vi "Frequency.vi"(8 "Samples per calculation":i32, 11 "Input waveform":waveform(dbl)) -> (3 "Frequency waveform":waveform(dbl))   [LabVIEW 2019]
uses:
  <vilib>/measure/mascope.llb/Pulse Measurements 1 chan.vi
  <vilib>/measure/NI_MAPro.lvlib
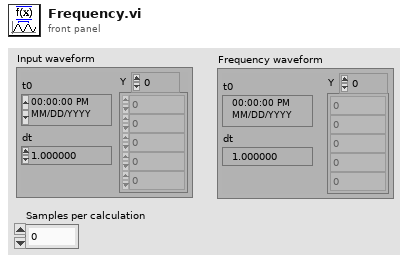
[diagram p1: front panel]
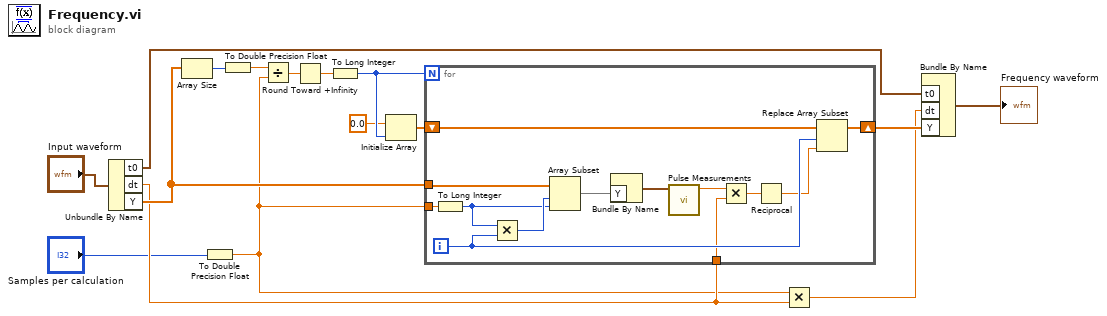
[diagram p0: block diagram]
diagram:
  n1 = Unbundle By Name("Input waveform") -> ("t0"=w5:timestamp, "dt"=w3:dbl, "Y"=w11:dbl[])
  n2 = Array Size(array=w11) -> (size(s)=w12:i32)
  n3 = To Double Precision Float(number="Samples per calculation") -> (double precision float=w1:dbl)
  n4 = To Double Precision Float(number=w12) -> (double precision float=w13:dbl)
  n5 = Divide(x=w13, y=w1) -> (x/y=w15:dbl)
  n6 = Round Toward +Infinity(x=w15) -> (ceil(x): smallest int >= x=w14:dbl)
  n7 = To Long Integer(number=w14) -> (32bit integer=w10:i32)
  n8 = Initialize Array(0.0 ("element"), w10) -> (w9:dbl[])
  n9 = for {
    N: w10 -> [_]
    tunnel: w11 -> [w28]
    tunnel: w1 -> [w26]
    shift-right: [w21] -> w6
    shift-left: w9 -> [w23]
    tunnel: w3 -> [w19]
    i -> [w22]
    n10 = To Long Integer(number=w26) -> (32bit integer=w24:i32)
    n11 = Multiply(x=w24, y=w22) -> (x*y=w25:i32)
    n12 = Array Subset(array=w28, index=w25, length=w24) -> (w27:dbl[])
    n13 = Bundle By Name("Y"=w27) -> (w29:waveform(dbl))  [unwired: 1 in]
    n14 = call-poly <vilib>:"Pulse Measurements.vi"("signal in"=w29) -> ("period"=w20:dbl)  [unwired: 6 in, 4 out]
    n15 = Multiply(x=w20, y=w19) -> (x*y=w18:dbl)
    n16 = Reciprocal(x=w18) -> (1/x=w17:dbl)
    n17 = Replace Array Subset(array=w23, new element=w17, index=w22) -> (w21:dbl[])
  }
  n18 = Multiply(x=w1, y=w3) -> (x*y=w4:dbl)
  n19 = Bundle By Name("t0"=w5, "dt"=w4, "Y"=w6) -> (→"Frequency waveform":waveform(dbl))  [unwired: 1 in]
